vi "SLSC Get Module Name (Cloned API).vi"(8 "error in (no error)":errorcluster, 11 "Item Ref in":T1 format="%.0x") -> (0 "error out":errorcluster, 2 "SLSC Module":string, 3 "Item Ref out":T1=18446744073709551615 format="%.0x")   [LabVIEW 2017]
uses:
  <vilib>/NI Veristand/Custom Device API/Custom Device Item Ref.ctl
  <vilib>/NI VeriStand/Custom Device API/Custom Device API.lvlib
panel:
  # "This VI is cloned from :\nC:\\Program Files (x86)\\National Instruments\\LabVIEW 2017\\vi.lib\\NI Veristand\\Custom Device API\\NI VeriStand - Get SLSC Module Name.vi\n\nUse this VI if you are using versions above 2017."
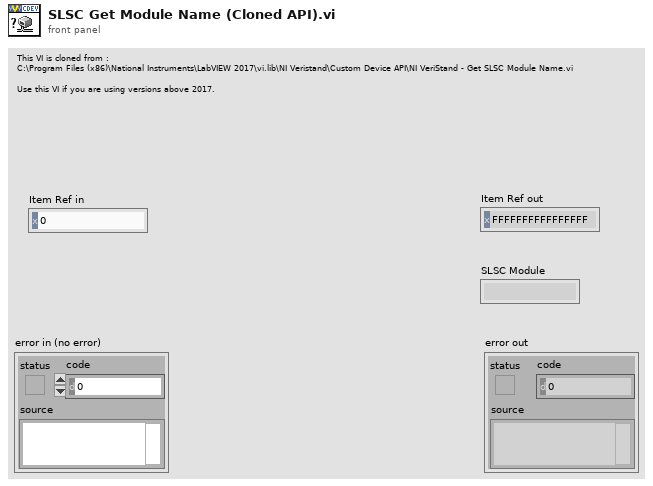
[diagram p1: front panel]
types:
  T1 = typedef "Custom Device API.lvlib/Custom Device Item Ref.ctl" = u64
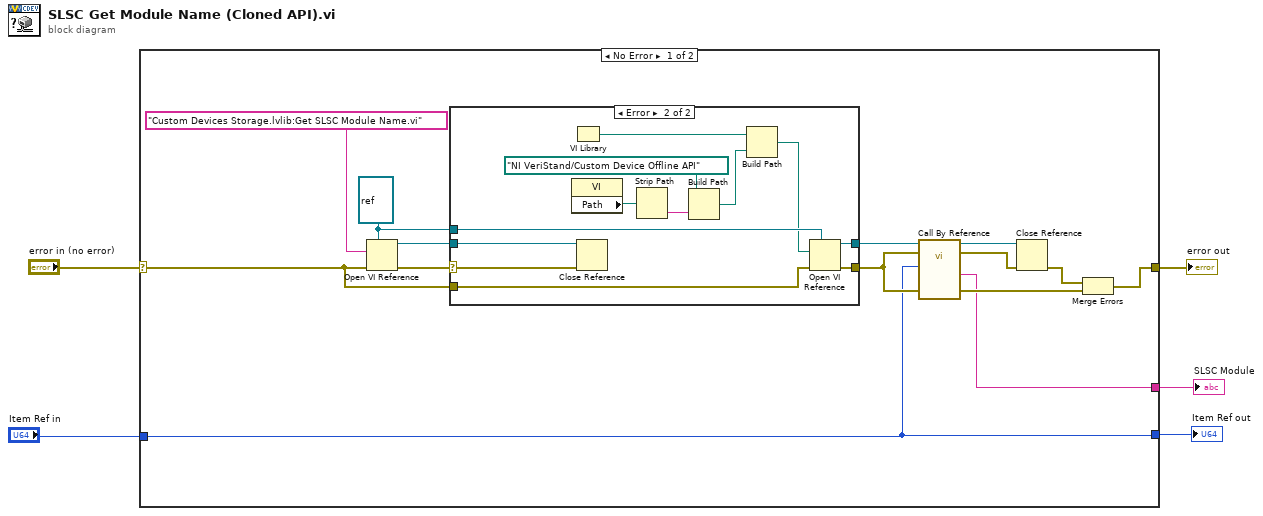
[diagram p0: block diagram]
diagram:
  n1 = case shown="No Error" "error in (no error)" {
    selector: "error in (no error)" -> [w7 w35]
    tunnel: [w14 w35] -> w5
    tunnel: [w8 _] -> w3
    tunnel: "Item Ref in" -> [w6 w34]
    tunnel: [w6 w34] -> w2
    frame No Error {
      w11 = refnum<vi> refnum ("type specifier VI Refnum (for type only)")
      n2 = Open VI Reference(type specifier VI Refnum (for type only)=w11, vi path="Custom Devices Storage.lvlib:Get SLSC Module Name.vi", error in (no error)=w7) -> (vi reference=w12:refnum<vi>, error out=w13:errorcluster)  [unwired: 3 out]
      n3 = case shown="Error" w13 {
        selector: w13 -> [w20 w30]
        tunnel: w11 -> [_ w32]
        tunnel: w12 -> [w21 w31]
        tunnel: [w21 w29] -> w10
        tunnel: [w20 w28] -> w9
        tunnel: w7 -> [_ w33]
        frame No Error {
        }
        frame Error {
          n4 = property class="VI"() -> ("Path"=w24:path)  [unwired: 2 in, 2 out]
          n5 = VI Library() -> (path=w27:path)
          n6 = Close Reference(reference=w31, error in (no error)=w30) -> ()  [unwired: 1 out]
          n7 = Strip Path(path=w24) -> (name=w23:string)  [unwired: 1 out]
          n8 = Build Path(base path=path "NI VeriStand/Custom Device Offline API", name or relative path=w23) -> (appended path=w26:path)
          n9 = Build Path(base path=w27, name or relative path=w26) -> (appended path=w25:path)
          n10 = Open VI Reference(type specifier VI Refnum (for type only)=w32, vi path=w25, error in (no error)=w33) -> (vi reference=w29:refnum<vi>, error out=w28:errorcluster)  [unwired: 3 out]
        }
      }
      n11 = call-by-ref "?"(reference=w10, error in=w9, 8:"error in (no error)"=w9, "Item Ref in"=w6) -> (reference out=w16:refnum<vi>, error out=w17:errorcluster, 0:"error out"=w18:errorcluster, "SLSC Module out"=w8:string)  [unwired: 8 in]
      n12 = Close Reference(reference=w16, error in (no error)=w17) -> (error out=w15:errorcluster)
      n13 = Merge Errors(w15, w18) -> (w14:errorcluster)
    }
    frame Error {
    }
  }
  "error out" <- w5
  "Item Ref out" <- w2
  "SLSC Module" <- w3
